vi "Is Clear.vi"(10 "Direction":T1, 11 "Maze (0: Empty, -1: Enemy. >0: Teammate in":i32[](array[numeric])) -> (3 "Is Clear":bool)   [LabVIEW 2020, in "Sentinel.lvclass"]
uses:
  Sentinel.lvclass
  Type Defs/Direction Enum.ctl
  Type Defs/SB Type Defs.lvlib
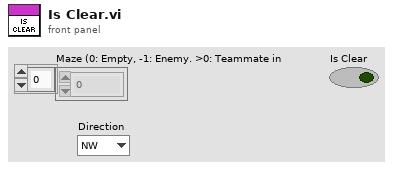
[diagram p1: front panel]
types:
  T1 = typedef "SB Type Defs.lvlib/Direction Enum.ctl" = enum16{"NW", "N", "NE", "E", "SE", "S", "SW", "W"}
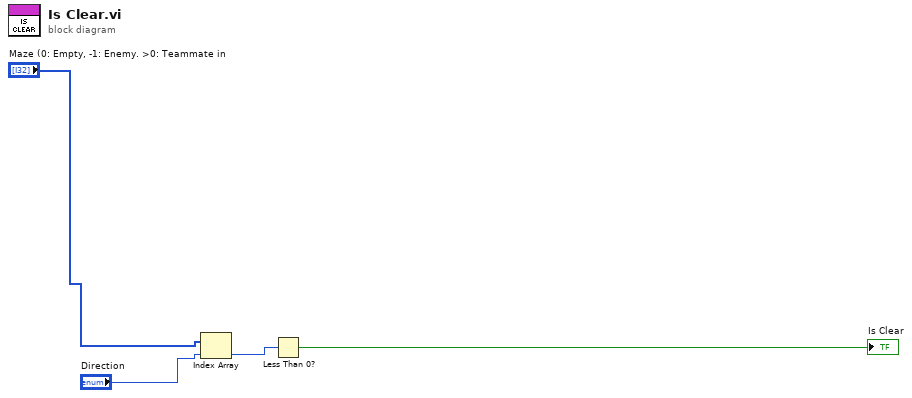
[diagram p0: block diagram]
diagram:
  n1 = Index Array(array="Maze (0: Empty, -1: Enemy. >0: Teammate in", index="Direction") -> (element=w2:i32)
  n2 = Less Than 0?(x=w2) -> (x < 0?=→"Is Clear":bool)
